vi "smooth speeed.vi"(10 "Numeric":dbl) -> (2 "Numeric 2":dbl)   [LabVIEW 2020]
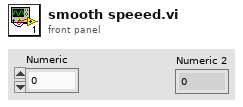
[diagram p1: front panel]
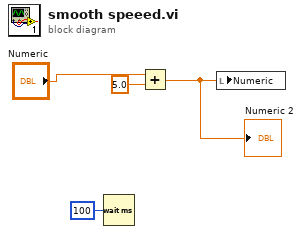
[diagram p0: block diagram]
diagram:
  n1 = Wait (ms)(milliseconds to wait=u32 100) -> ()  [unwired: 1 out]
  n2 = Add(x="Numeric", y=5.0) -> (x+y=w2:dbl)
  "Numeric 2" <- w2
  n3 = local write "Numeric"(w2) -> ()
